vi "NumIntegrate_Func_Bs.vi"(9 "Col":i32, 11 "Row":i32) -> (3 "Bs":dbl)   [LabVIEW 2019, in "Trajectory_Library.lvlib"]
doc: "Internal function used by Rkf45_Impl.vi\n\nInputs:\n - Row -- Row to look up ( 0 - 5 )\n - Column -- Column value to look up ( 0 - 4 )\n\nOutputs:\n - Bs -- Value looked up by index."
uses:
  Trajectory_Library.lvlib
  <vilib>/Analysis/Matrix/Datatypes/RealMatrix.ctl
  <vilib>/Analysis/Matrix/NI_Matrix.lvlib
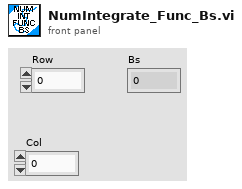
[diagram p1: front panel]
types:
  T1 = typedef "NI_Matrix.lvlib/RealMatrix.ctl" = dbl[][]
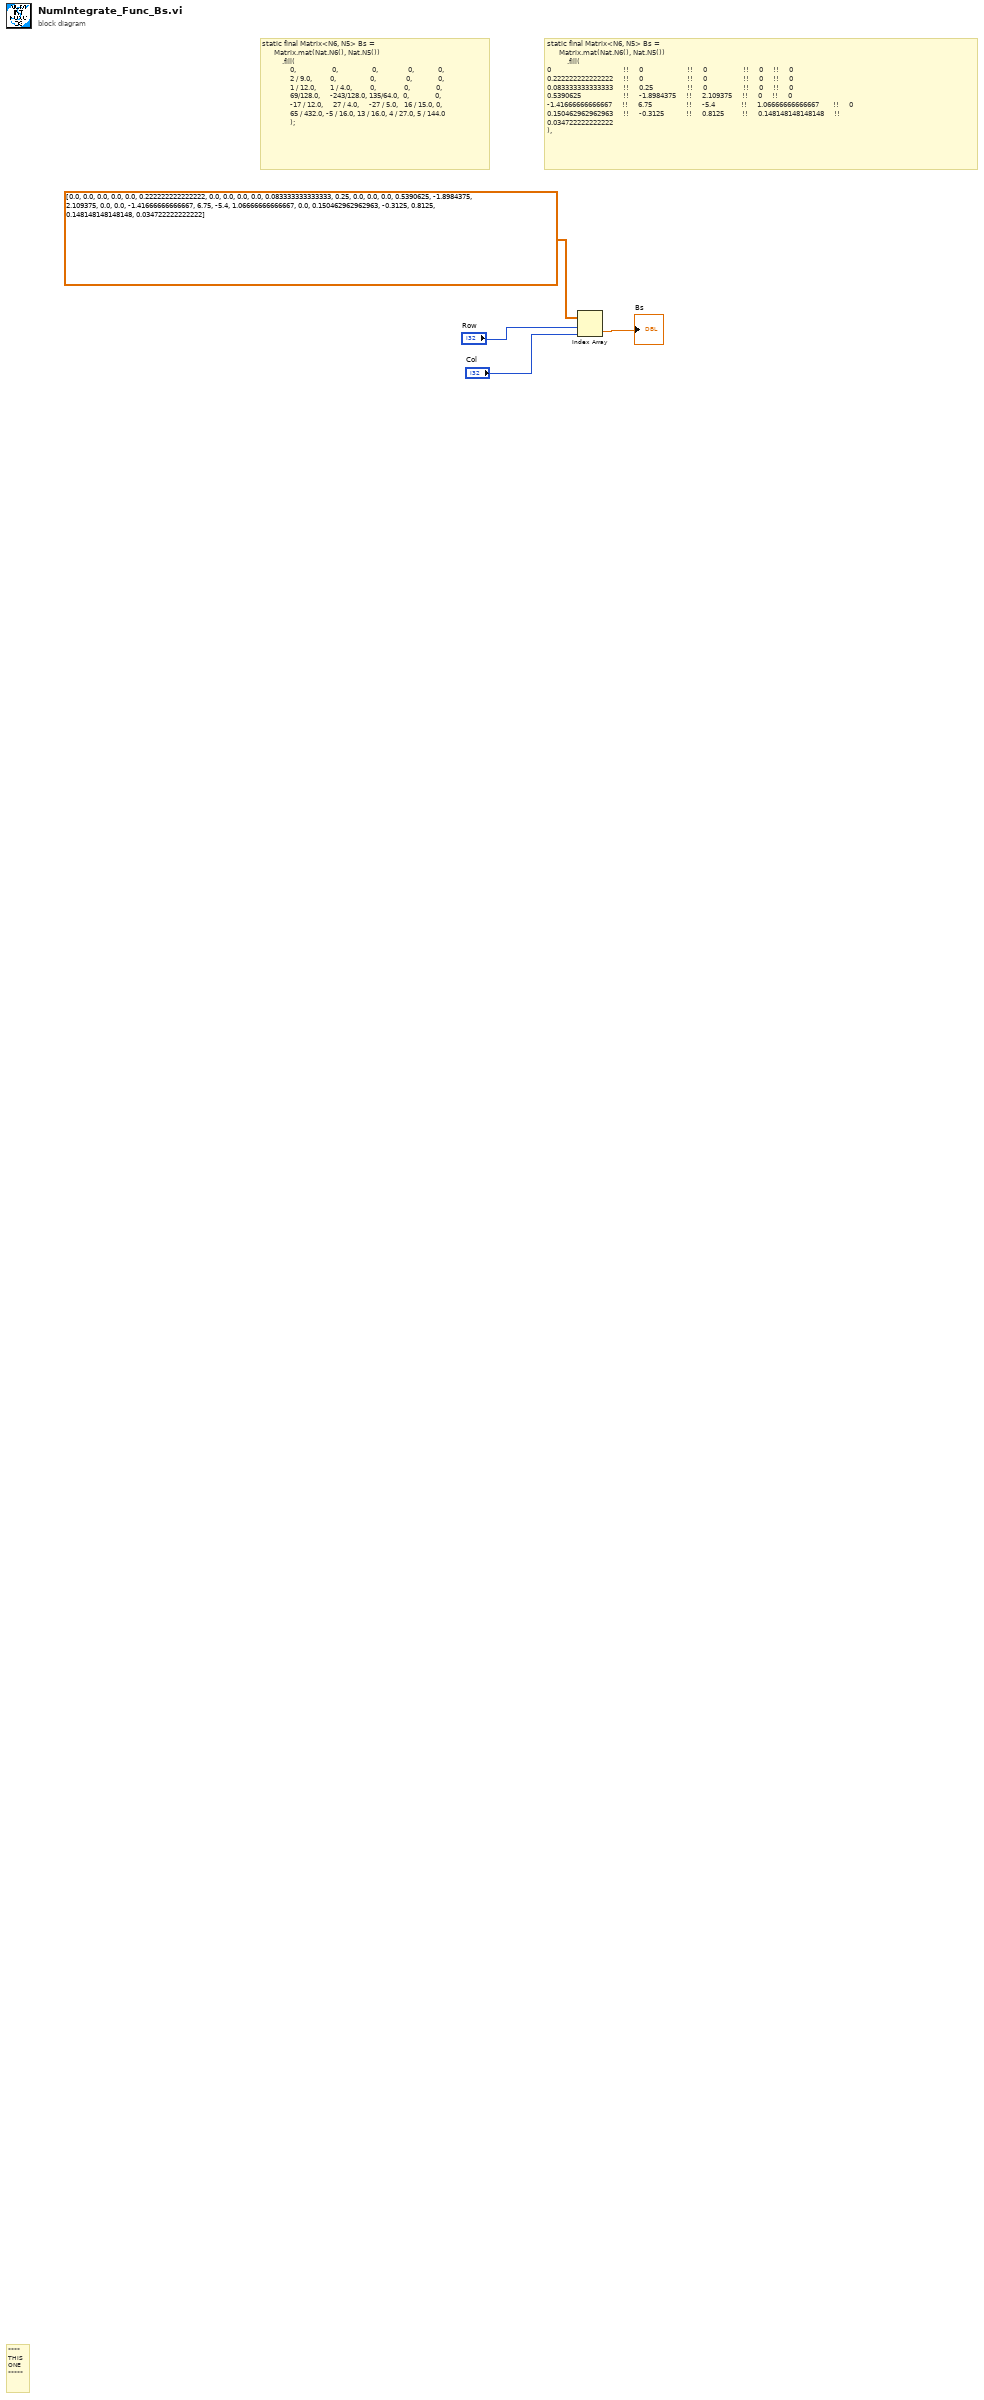
[diagram p0: block diagram]
diagram:
  # "static final Matrix<N6, N5> Bs =\t\t\t\t\t\t\t\t\n      Matrix.mat(Nat.N6(), Nat.N5())\t\t\t\t\t\t\t\t\n          .fill(\t\t\t\t\t\t\t\t\n0\t                                   !!    \t0\t                     !!    \t0\t                 !!    \t0\t    !!    \t0\n0.222222222222222\t    !!    \t0\t                     !!    \t0\t                 !!    \t0\t    !!    \t0\n0.083333333333333\t    !!    \t0.25\t                !!    \t0\t                 !!    \t0\t    !!    \t0\n0.5390625\t                    !!    \t-1.8984375\t    !!    \t2.109375\t    !!    \t0\t    !!    \t0\n-1.41666666666667\t    !!    \t6.75\t                !!    \t-5.4\t            !!    \t1.06666666666667\t      !!    \t0\n0.150462962962963\t    !!    \t-0.3125\t          !!    \t0.8125\t        !!    \t0.148148148148148\t    !!    \t0.034722222222222\n),"
  # "static final Matrix<N6, N5> Bs =\n      Matrix.mat(Nat.N6(), Nat.N5())\n          .fill(\n              0,\t                 0,\t                0,\t              0,\t           0,\n              2 / 9.0,\t        0,\t                0,\t              0,\t            0,\n              1 / 12.0,\t      1 / 4.0,         0,\t             0,\t            0,\t\n              69/128.0,     -243/128.0, 135/64.0,  0,             0,\n              -17 / 12.0,     27 / 4.0,     -27 / 5.0,   16 / 15.0, 0,\n              65 / 432.0, -5 / 16.0, 13 / 16.0, 4 / 27.0, 5 / 144.0\n              );"
  # "****\nTHIS\nONE\n*****"
  n1 = Index Array(array=T1 [[0.0, 0.0, 0.0, 0.0, 0.0], [0.222222222222222, 0.0, 0.0, 0.0, 0.0], [0.083333333333333, 0.25, 0.0, 0.0, 0.0], [0.5390625, -1.8984375, 2.109375, 0.0, 0.0], [-1.41666666666667, 6.75, -5.4, 1.06666666666667, 0.0], [0.150462962962963, -0.3125, 0.8125, 0.148148148148148, 0.034722222222222]] ("matrix"), index (row)="Row", index (col)="Col") -> (element=→"Bs":dbl)
